vi "Last Error to Wire.vi"(2 "MultiErrors in":refnum<class "MultiErrors.lvclass">) -> (7 "error out":errorcluster)   [LabVIEW 2020, in "VolatusErrorUtilities.lvlib" / "MultiErrors.lvclass"]
uses:
  MultiErrors.lvclass
  MultiErrors.lvclass/MultiErrors.ctl
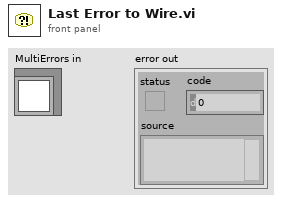
[diagram p1: front panel]
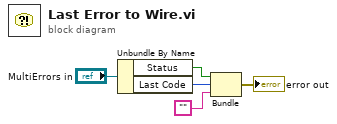
[diagram p0: block diagram]
diagram:
  n1 = Unbundle By Name("MultiErrors in") -> ("Status"=w4:bool, "Last Code"=w3:i32)
  n2 = Bundle("Status"=w4, "Last Code"=w3, "") -> (→"error out":cluster{"Status":bool, "Last Code":i32, string})  [unwired: 1 in]
